vi "Documentation Application Tool.vi"() -> ()   [LabVIEW 2016]
uses:
  <vilib>/xml/NI_XML.lvlib
  <resource>/objmgr/DOMUserDefRef.rc
panel:
  out "Local Name":string
  out "Parse Errors":string
  in  "Load XML File":bool
  in  "XML File Path":path
  in  "Load Search Directory":bool
  in  "Search Directory":path
  in  "Code Modules":string(tree)
  in  "Description":string
  in  "Copy":bool
  out "Matched XML Data":string
  in  "XML XPath Query":string
  in  "Apply":bool
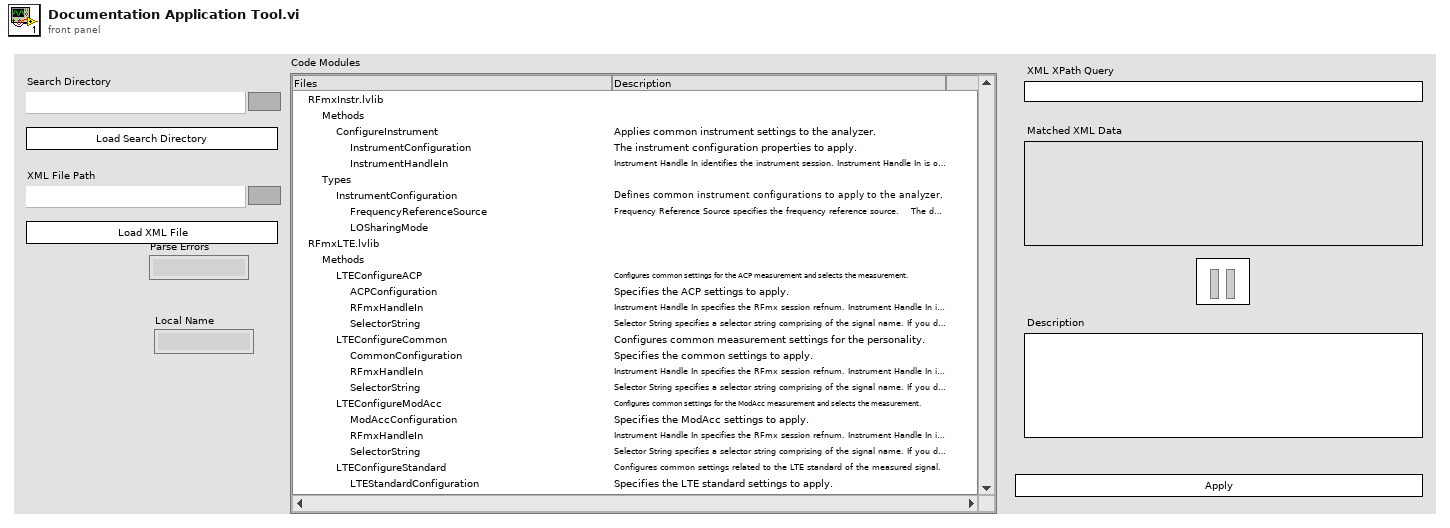
[diagram p1: front panel]
types:
  T1 = enum32{"invalid VI type", "Standard VI", "Control VI", "Global VI", "Polymorphic VI", "Configuration VI", "SubSystem", "Facade VI", "Method VI", "Statechart Diagram VI"}
  T2 = enum8{"Enabled", "Disabled", "Disabled and Grayed Out"}
  T3 = cluster{enum16{"VI", "Control"}, "Variant":variant}
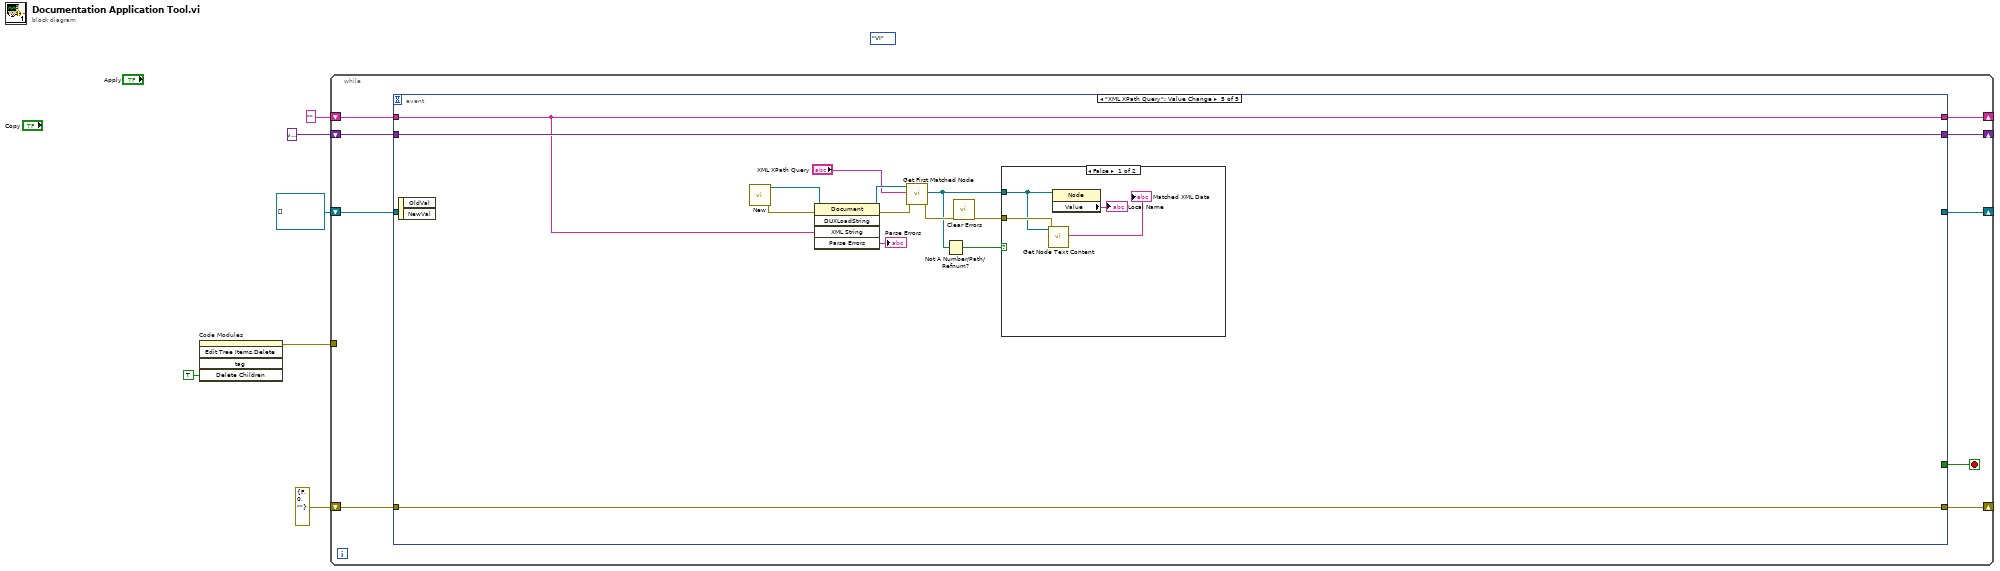
[diagram p0: block diagram]
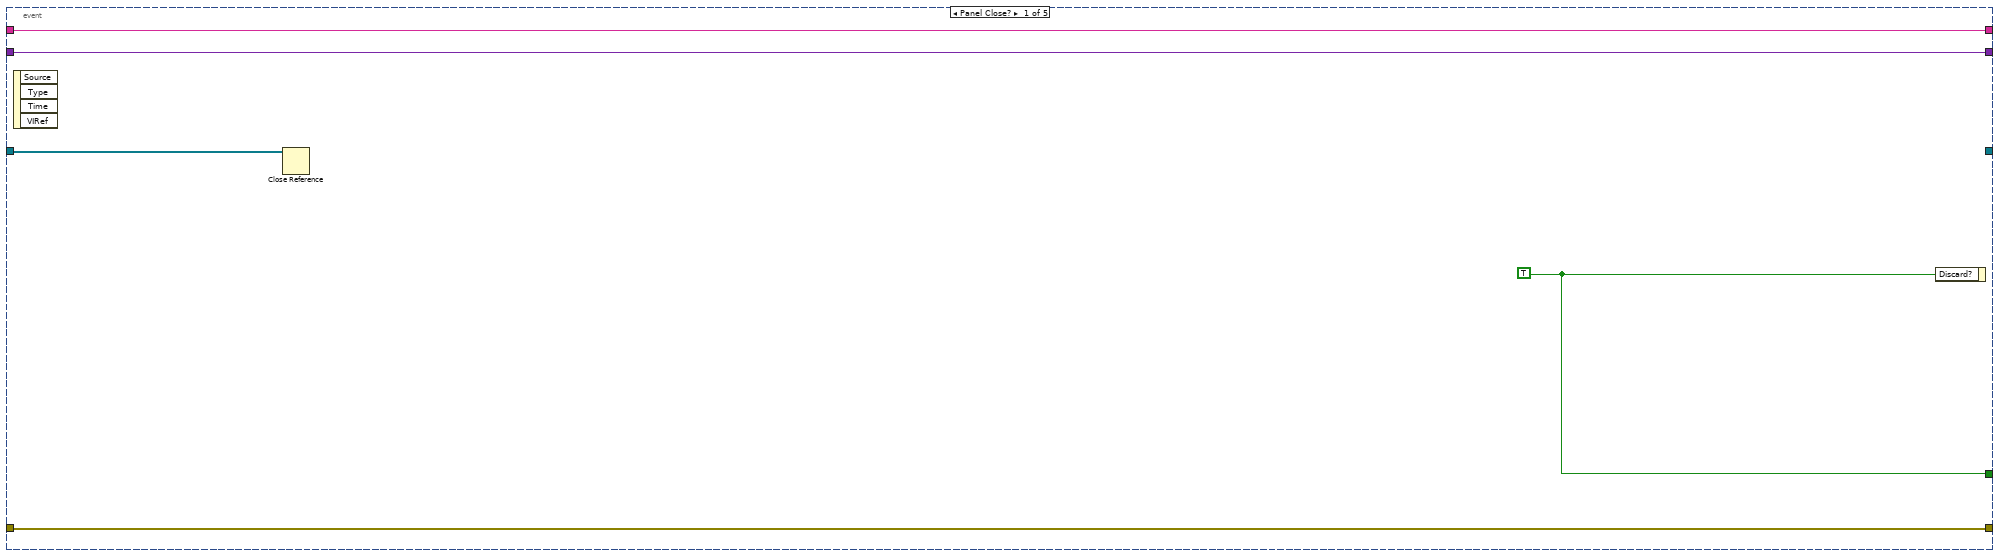
[diagram p2: hidden frame]
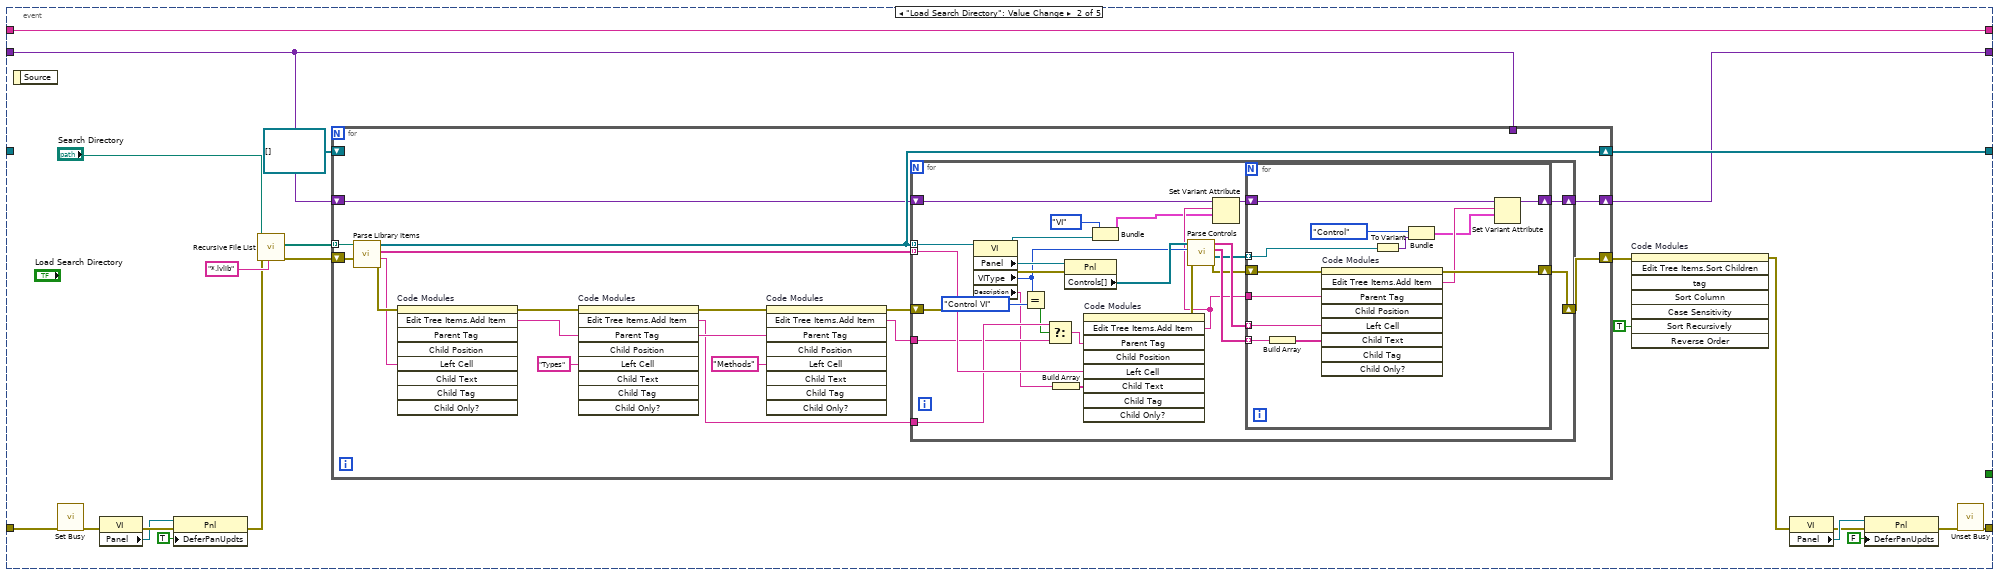
[diagram p3: hidden frame]
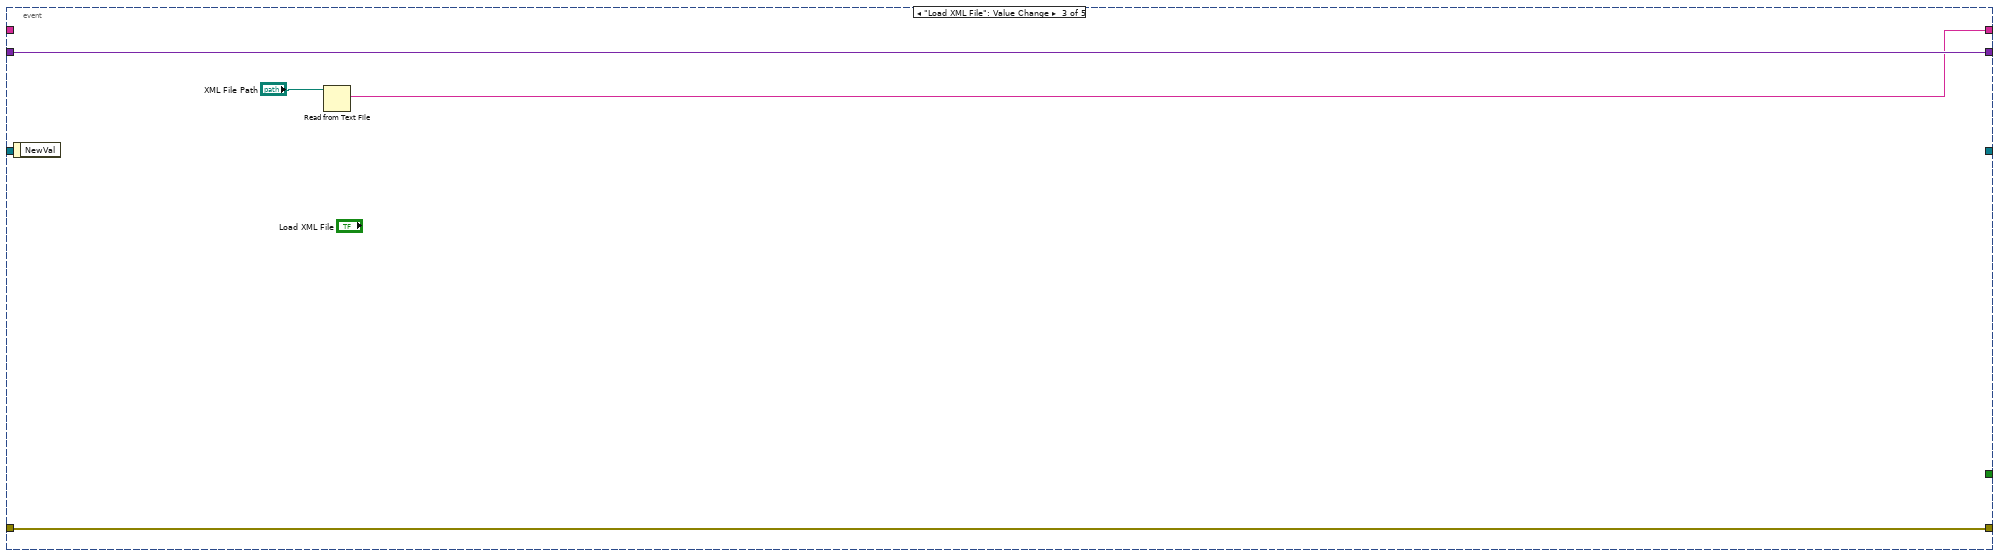
[diagram p4: hidden frame]
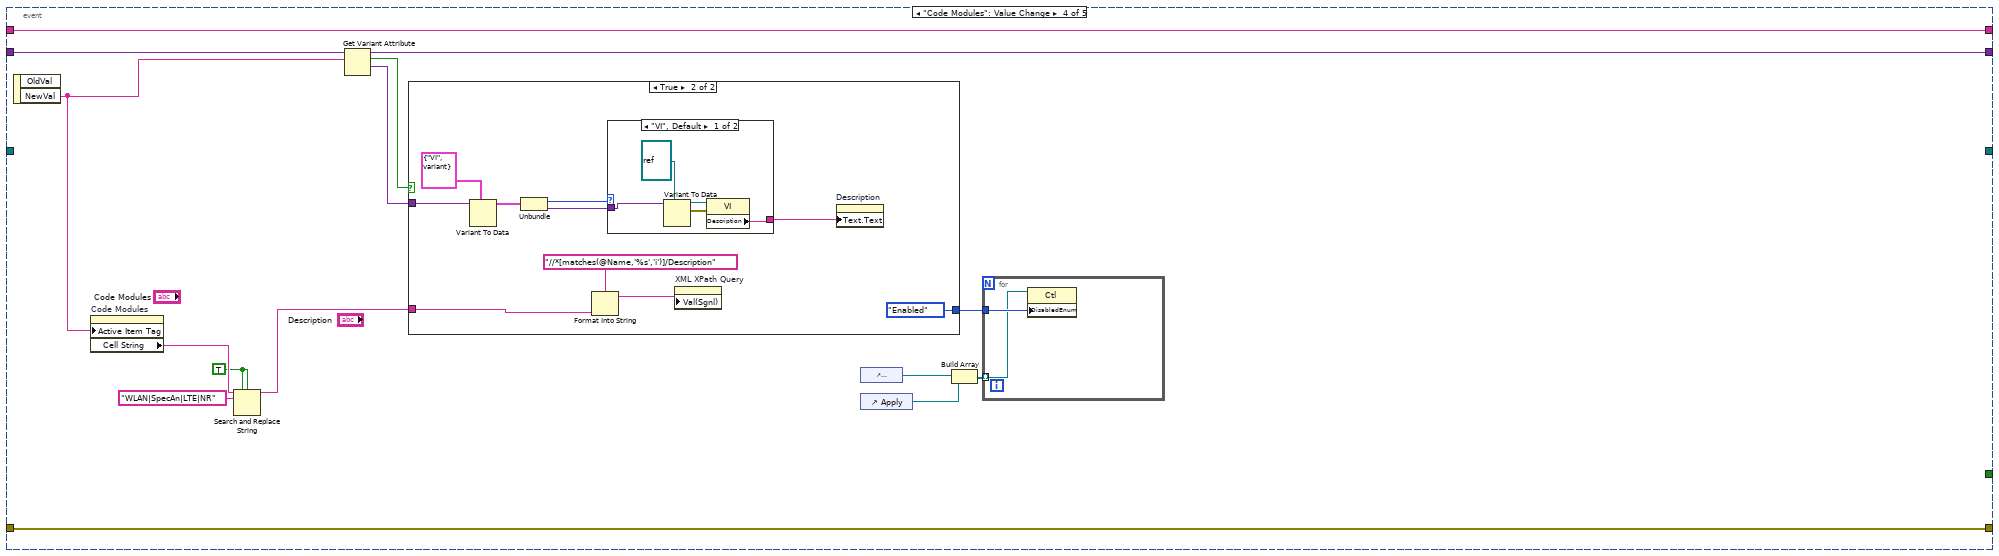
[diagram p5: hidden frame]
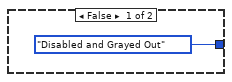
[diagram p6: hidden frame]
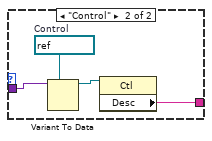
[diagram p7: hidden frame]
diagram:
  (unwired) enum16{"VI", "Control"}."VI"
  n1 = invoke on="Code Modules" class="Tree (strict)" method="Edit Tree Items.Delete"("Delete Children"=TRUE ("Delete Children?")) -> (error out=w4:errorcluster)  [unwired: 4 in, 4 out]
  n2 = while {
    shift-right: [w14] -> _
    shift-left: errorcluster {"status"=FALSE, "code"=0, "source"=""} ("error constant") -> [w15]
    shift-right: [w12] -> _
    shift-left: refnum<vi>[] [] ("References") -> [w11]
    tunnel: w4 -> [_]
    shift-right: [w10] -> _
    shift-left: variant -> [w9]
    shift-right: [w7] -> _
    shift-left: "" -> [w8]
    stop <- w13 stop-if-true
    n3 = event shown="[4] \"XML XPath Query\": Value Change" {
      selector: _ -> [_ _ _ _ _]
      dyn-events: _ -> [_ _ _ _ _]
      timeout: _ -> [_ _ _ _ _]
      tunnel: [w19 _ _ _ _] -> w13
      tunnel: w15 -> [w20 w42 w102 w117 w152]
      tunnel: [w20 w35 w102 w117 w152] -> w14
      tunnel: [_ w37 _ _ _] -> w12
      tunnel: w11 -> [w18 _ _ _ _]
      tunnel: [w17 w22 w101 w115 w151] -> w10
      tunnel: w9 -> [w17 w23 w101 w116 w151]
      tunnel: w8 -> [w16 w21 _ w108 w149]
      tunnel: [w16 w21 w99 w108 w149] -> w7
      event Panel Close? {
        w19 = TRUE ("Discard?")
        n4 = event-data() -> ()  [unwired: 1 in, 4 out]
        n5 = Close Reference(reference=w18) -> ()  [unwired: 1 in, 1 out]
        n6 = event-data("Discard?"=w19) -> ()  [unwired: 1 in, 1 out]
      }
      event "Load Search Directory": Value Change {
        n7 = event-data() -> ()  [unwired: 1 in, 1 out]
        n8 = call <vilib>:"Set Busy.vi"("error in (no error)"=w42) -> ("error out"=w36:errorcluster)  [unwired: 9 in, 1 out]
        n9 = property class="VI"(error in=w36) -> (error out=w34:errorcluster, "Panel"=w32:refnum<vi>)  [unwired: 1 in, 1 out]
        n10 = property class="Pnl"(reference=w32, error in=w34, "DeferPanUpdts"=TRUE ("Defer Panel Updates")) -> (error out=w33:errorcluster)  [unwired: 1 out]
        n11 = call <vilib>:"Recursive File List.vi"("pattern"="*.lvlib", "error in (no error)"=w33, "Folder Path"="Search Directory") -> ("error out"=w43:errorcluster, "All Files in Dir"=w39:path[])  [unwired: 4 in, 3 out]
        n12 = for {
          tunnel: w39 -> [w57] mode=indexing
          shift-right: [w55] -> w37
          shift-left: refnum<vi>[] [] ("References") -> [_]
          shift-right: [w52] -> w26
          shift-left: w43 -> [w58]
          tunnel: w23 -> [_]
          shift-right: [w44] -> w22
          shift-left: w23 -> [w45]
          n13 = call "Parse Library Items.vi"("error in (no error)"=w58, "Library Path"=w57) -> ("error out"=w54:errorcluster, "Display Name"=w50:string, "File Names"=w56:string[], "References"=w55:refnum<vi>[])  [unwired: 6 in]
          n14 = invoke on="Code Modules" class="Tree (strict)" method="Edit Tree Items.Add Item"(error in=w54, "Left Cell"=w50) -> (error out=w53:errorcluster, "Edit Tree Items:Add Item"=w48:string)  [unwired: 7 in, 7 out]
          n15 = invoke on="Code Modules" class="Tree (strict)" method="Edit Tree Items.Add Item"("Parent Tag"=w48, "Left Cell"="Types" ("Left Cell String")) -> ("Edit Tree Items:Add Item"=w47:string)  [unwired: 7 in, 8 out]
          n16 = invoke on="Code Modules" class="Tree (strict)" method="Edit Tree Items.Add Item"("Parent Tag"=w48, "Left Cell"="Methods" ("Left Cell String")) -> ("Edit Tree Items:Add Item"=w46:string)  [unwired: 7 in, 8 out]
          n17 = for {
            tunnel: w55 -> [w85] mode=indexing
            tunnel: w56 -> [w84] mode=indexing
            shift-right: [w67] -> w52
            shift-left: w53 -> [w83]
            tunnel: w47 -> [w79]
            tunnel: w46 -> [w78]
            shift-right: [w65] -> w44
            shift-left: w45 -> [w64]
            n18 = property class="VI"(reference=w85, error in=w83) -> (reference out=w60:refnum<vi>, error out=w82:errorcluster, "Panel"=w81:refnum<vi>, "VIType"=w74:T1, "Description"=w71:string)
            n19 = Equal?(x=w74, y=T1."Control VI") -> (x = y?=w77:bool)
            n20 = Select(t=w79, s=w77, f=w78) -> (s? t:f=w76:string)
            n21 = Build Array(w71) -> (w70:string[])
            n22 = property class="Pnl"(reference=w81, error in=w82) -> ("Controls[]"=w75:refnum<vi>[])  [unwired: 2 out]
            n23 = invoke on="Code Modules" class="Tree (strict)" method="Edit Tree Items.Add Item"("Parent Tag"=w76, "Left Cell"=w84, "Child Text"=w70) -> (error out=w68:errorcluster, "Edit Tree Items:Add Item"=w62:string)  [unwired: 6 in, 7 out]
            n24 = Bundle(enum16{"VI", "Control"}."VI", w60) -> (w59:cluster{enum16{"VI", "Control"}, refnum<vi>})  [unwired: 1 in]
            n25 = call "Parse Controls.vi"("error in (no error)"=w68, "VI Type"=w74, "Controls[]"=w75) -> ("error out"=w69:errorcluster, "References"=w66:refnum<vi>[], "Control Descriptions"=w72:string[], "Control Names"=w73:string[])  [unwired: 5 in]
            n26 = Set Variant Attribute(Variant=w64, name=w62, value=w59) -> (Variant out=w63:variant)  [unwired: 1 in, 2 out]
            n27 = for {
              tunnel: w73 -> [w98] mode=indexing
              tunnel: w72 -> [w97] mode=indexing
              tunnel: w62 -> [w95]
              shift-right: [w93] -> w67
              shift-left: w69 -> [w94]
              tunnel: w66 -> [w89] mode=indexing
              shift-right: [w91] -> w65
              shift-left: w63 -> [w92]
              n28 = Build Array(w97) -> (w96:string[])
              n29 = invoke on="Code Modules" class="Tree (strict)" method="Edit Tree Items.Add Item"(error in=w94, "Parent Tag"=w95, "Left Cell"=w98, "Child Text"=w96) -> (error out=w93:errorcluster, "Edit Tree Items:Add Item"=w90:string)  [unwired: 5 in, 7 out]
              n30 = To Variant(anything=w89) -> (Variant=w87:variant)
              n31 = Bundle(enum16{"VI", "Control"}."Control", "Variant"=w87) -> (w86:T3)  [unwired: 1 in]
              n32 = Set Variant Attribute(Variant=w92, name=w90, value=w86) -> (Variant out=w91:variant)  [unwired: 1 in, 2 out]
            }
          }
        }
        n33 = invoke on="Code Modules" class="Tree (strict)" method="Edit Tree Items.Sort Children"(error in=w26, "Sort Recursively"=TRUE ("Sort Recursively?")) -> (error out=w25:errorcluster)  [unwired: 6 in, 7 out]
        n34 = property class="VI"(error in=w25) -> (error out=w28:errorcluster, "Panel"=w29:refnum<vi>)  [unwired: 1 in, 1 out]
        n35 = property class="Pnl"(reference=w29, error in=w28, "DeferPanUpdts"=FALSE ("Defer Panel Updates")) -> (error out=w27:errorcluster)  [unwired: 1 out]
        n36 = call <vilib>:"Unset Busy.vi"("error in (no error)"=w27) -> ("error out"=w35:errorcluster)  [unwired: 10 in]
      }
      event "Load XML File": Value Change {
        n37 = event-data() -> ()  [unwired: 1 in, 1 out]
        n38 = Read from Text File(file (use dialog)="XML File Path") -> (text=w99:string)  [unwired: 3 in, 3 out]
      }
      event "Code Modules": Value Change {
        w103 = TRUE ("replace all? (F)")
        n39 = event-data() -> ("NewVal"=w107:string)  [unwired: 1 in, 1 out]
        n40 = property on="Code Modules" class="Tree (strict)"("Active Item Tag"=w107) -> ("Cell String"=w106:string)  [unwired: 2 in, 2 out]
        n41 = Search and Replace String(replace all?=w103, case sensitive?=w103, input string=w106, search string="WLAN|SpecAn|LTE|NR") -> (result string=w105:string)  [unwired: 4 in, 3 out]
        n42 = Get Variant Attribute(Variant=w116, name=w107) -> (duplicate Variant=w115:variant, found=w113:bool, value=w114:variant)  [unwired: 2 in, 1 out]
        n43 = case shown="True" w113 {
          tunnel: w114 -> [_ w129]
          tunnel: [T2."Disabled and Grayed Out" ("Disabled") T2."Enabled" ("Disabled")] -> w112
          tunnel: w105 -> [_ w122]
          frame False {
          }
          frame True {
            n44 = Variant To Data(type=T3 {enum."VI", "Variant"=variant} ("cluster"), Variant=w129) -> (data=w127:T3)  [unwired: 1 in, 1 out]
            n45 = Unbundle(w127) -> (w126:enum16{"VI", "Control"}, "Variant"=w125:variant)
            n46 = Format Into String(format string="//*[matches(@Name,'%s','i')]/Description", w122) -> (resulting string=w121:string)  [unwired: 2 in, 1 out]
            n47 = case shown="\"VI\", Default" w126 {
              tunnel: [w131 w137] -> w130
              tunnel: w125 -> [w135 w136]
              frame "VI", Default {
                n48 = Variant To Data(type=refnum<vi> refnum ("vi reference"), Variant=w135) -> (data=w133:refnum<vi>, error out=w132:errorcluster)  [unwired: 1 in]
                n49 = property class="VI"(reference=w133, error in=w132) -> ("Description"=w131:string)  [unwired: 2 out]
              }
              frame "Control" {
                w139 = refnum<vi> refnum  # Control
                n50 = Variant To Data(type=w139, Variant=w136) -> (data=w138:refnum<vi>)  [unwired: 1 in, 1 out]
                n51 = property class="Ctl"(reference=w138) -> ("Desc"=w137:string)  [unwired: 1 in, 2 out]
              }
            }
            n52 = property on="XML XPath Query" class="Str"("Val(Sgnl)"=w121) -> ()  [unwired: 2 in, 2 out]
            n53 = property on="Description" class="Str"("Text.Text"=w130) -> ()  [unwired: 2 in, 2 out]
          }
        }
        n54 = control-ref of="Description"() -> (w111:refnum<vi>)
        n55 = control-ref of="Apply"() -> (w110:refnum<vi>)
        n56 = Build Array(w111, w110) -> (w109:refnum<vi>[])
        n57 = for {
          tunnel: w112 -> [w119]
          tunnel: w109 -> [w118] mode=indexing
          n58 = property class="Ctl"(reference=w118, "DisabledEnum"=w119) -> ()  [unwired: 1 in, 2 out]
        }
      }
      event "XML XPath Query": Value Change {
        n59 = event-data() -> ()  [unwired: 1 in, 2 out]
        n60 = call <vilib>:"New.vi"() -> ("error out"=w146:errorcluster, "DOM document out"=w150:refnum<k20>)  [unwired: 8 in]
        n61 = invoke class="Document" method="DUXLoadString"(reference=w150, error in=w146, "XML String"=w149) -> (reference out=w148:refnum<k20>, error out=w145:errorcluster, "Parse Errors"=→"Parse Errors":string)  [unwired: 2 in, 2 out]
        n62 = call <vilib>:"Get First Matched Node.vi"("error in (no error)"=w145, "XPath expression"="XML XPath Query", "node in"=w148) -> ("error out"=w143:errorcluster, "node result"=w140:refnum<k20>)  [unwired: 6 in, 1 out]
        n63 = Not A Number/Path/Refnum?(number/path/refnum=w140) -> (NaN/Path/Refnum?=w144:bool)
        n64 = call <vilib>:"Clear Errors.vi"("error in (no error)"=w143) -> ("error out"=w142:errorcluster)  [unwired: 5 in, 1 out]
        n65 = case shown="False" w144 {
          tunnel: w142 -> [w155 _]
          tunnel: w140 -> [w153 _]
          frame False {
            n66 = call <vilib>:"Get Node Text Content.vi"("error in (no error)"=w155, "node in"=w153) -> ("node text"=→"Matched XML Data":string)  [unwired: 7 in, 2 out]
            n67 = property class="Node"(reference=w153) -> ("Value"=→"Local Name":string)  [unwired: 1 in, 2 out]
          }
          frame True {
          }
        }
      }
    }
  }
